vi "Test Enr tdms.vi"() -> ()   [LabVIEW 2021]
panel:
  out "Graphe":dbl[](graph)
  in  "stop":bool
  out "chemin complet":path
  in  "Chemin du fichier":path
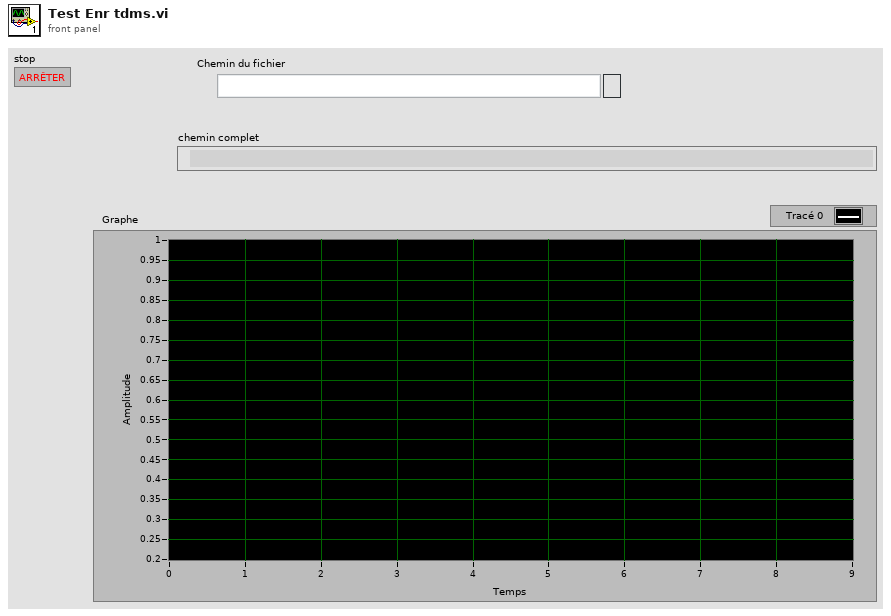
[diagram p1: front panel]
types:
  T1 = cluster{"Waveform":waveform(dbl)[], "Delta_tps":timestamp[], "time":string[]}
  T2 = enum16{"open", "open or create", "create or replace", "create", "open (read-only)"}
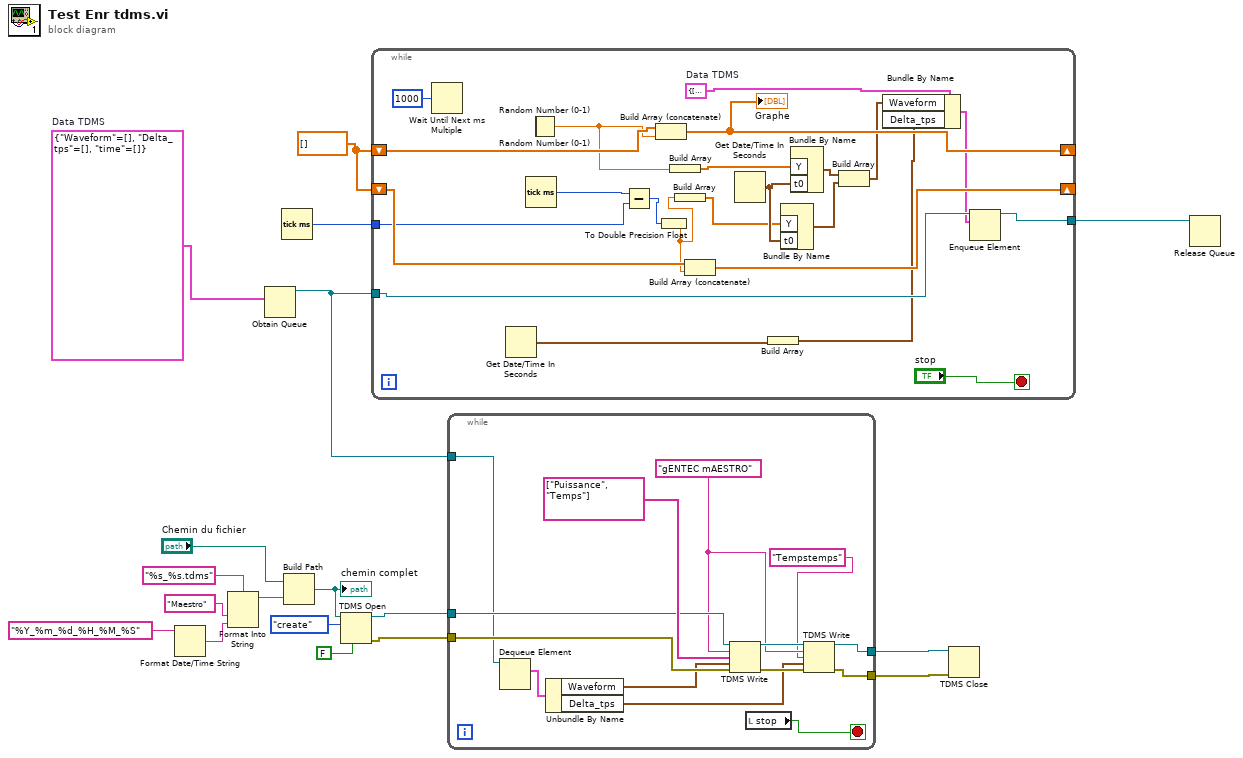
[diagram p0: block diagram]
diagram:
  w1 = T1 {"Waveform"=[], "Delta_tps"=[], "time"=[]}  # Data TDMS
  w4 = dbl[] []
  n1 = Format Date/Time String(time format string (%c)="%Y_%m_%d_%H_%M_%S") -> (date/time string=w15:string)  [unwired: 2 in]
  n2 = Format Into String(format string="%s_%s.tdms", "Maestro" ("entrée 1"), w15) -> (resulting string=w17:string)  [unwired: 2 in, 1 out]
  n3 = Obtain Queue(element data type=w1) -> (queue out=w5:refnum<queue>)  [unwired: 4 in, 2 out]
  n4 = Tick Count (ms)() -> (millisecond timer value=w3:u32)
  n5 = Build Path(base path="Chemin du fichier", name or relative path=w17) -> (appended path=w14:path)
  "chemin complet" <- w14
  n6 = TDMS Open(6:FALSE ("désactiver la bufférisation ? (V)"), 10:T2."create" ("opération (0 : open)"), 11:w14) -> (0:w9:errorcluster, 3:w8:refnum<k34>)  [unwired: 4 in]
  n7 = while {
    tunnel: w5 -> [w36]
    tunnel: [w35] -> w18
    shift-right: [w28] -> _
    shift-left: w4 -> [w32]
    shift-right: [w30] -> _
    shift-left: w4 -> [w31]
    tunnel: w3 -> [w29]
    stop <- "stop" stop-if-true
    w21 = T1 {"Waveform"=[], "Delta_tps"=[], "time"=[]}  # Data TDMS
    n8 = Wait Until Next ms Multiple(millisecond multiple=u32 1000 ("n millisecondes")) -> ()  [unwired: 1 out]
    n9 = Get Date/Time In Seconds() -> (seconds since 1Jan1904=w20:timestamp)
    n10 = Tick Count (ms)() -> (millisecond timer value=w33:u32)
    n11 = Random Number (0-1)() -> (number: 0 to 1=w27:dbl)
    n12 = Random Number (0-1)() -> ()  [unwired: 1 out]
    n13 = Subtract(x=w33, y=w29) -> (x-y=w39:u32)
    n14 = Build Array (concatenate)(w32, w27) -> (w28:dbl[])
    "Graphe" <- w28
    n15 = To Double Precision Float(number=w39) -> (double precision float=w25:dbl)
    n16 = Build Array(w27) -> (w26:dbl[])
    n17 = Build Array(w25) -> (w24:dbl[])
    n18 = Build Array (concatenate)(w31, w25) -> (w30:dbl[])
    n19 = Get Date/Time In Seconds() -> (seconds since 1Jan1904=w40:timestamp)
    n20 = Build Array(w20) -> (w19:timestamp[])
    n21 = Bundle By Name("Y"=w24, "t0"=w40) -> (w38:waveform(dbl))  [unwired: 1 in]
    n22 = Bundle By Name("Y"=w26, "t0"=w40) -> (w41:waveform(dbl))  [unwired: 1 in]
    n23 = Build Array(w41, w38) -> (w23:waveform(dbl)[])
    n24 = Bundle By Name(cluster=w21, "Waveform"=w23, "Delta_tps"=w19) -> (w22:T1)
    n25 = Enqueue Element(queue=w36, element=w22) -> (queue out=w35:refnum<queue>)  [unwired: 2 in, 2 out]
  }
  n26 = while {
    tunnel: w9 -> [w54]
    tunnel: w8 -> [w53]
    tunnel: [w47] -> w7
    tunnel: [w49] -> w6
    tunnel: w5 -> [w51]
    stop <- w52 stop-if-true
    w46 = "gENTEC mAESTRO" ("nom du groupe en entrée (Sans titre)")
    n27 = Dequeue Element(queue=w51) -> (element=w45:T1)  [unwired: 2 in, 3 out]
    n28 = Unbundle By Name(w45) -> ("Waveform"=w44:waveform(dbl)[], "Delta_tps"=w43:timestamp[])
    n29 = TDMS Write(0:w53, 5:w46, 7:string[] ["Puissance", "Temps"] ("nom des voies en entrée (Sans titre)"), 9:w44, 11:w54) -> (4:w50:refnum<k34>, 15:w48:errorcluster)  [unwired: 1 in, 2 out]
    n30 = local read "stop"() -> (w52:bool)
    n31 = TDMS Write(0:w50, 5:w46, 7:"Tempstemps", 9:w43, 11:w48) -> (4:w49:refnum<k34>, 15:w47:errorcluster)  [unwired: 1 in, 2 out]
  }
  n32 = TDMS Close(8:w7, 11:w6) -> ()  [unwired: 2 out]
  n33 = Release Queue(queue=w18) -> ()  [unwired: 2 in, 3 out]
